vi "SENS_AVER.vi"(0 "VISA IN":refnum<visa-resource-name>, 2 "Average ON/OFF":bool, 5 "error in":errorcluster, 7 "Channel":i32) -> (14 "VISA Out":refnum<visa-resource-name>, 19 "error out":errorcluster)   [LabVIEW 2018, in "PNA-X.lvlib"]
doc: "SENSe<cnum>:AVERage:CLEar \n(Write-only) Clears and restarts averaging of the measurement data. Must also set \nSENS:AVER[:STATe] ON \nParameters \n<cnum> Any existing channel number; if unspecified, value is set to 1. \nExamples SENS:AVER:CLE \nsense2:average:clear \nQuery Syntax Not applicable \nDefault Not applicable"
uses:
  PNA-X.lvlib
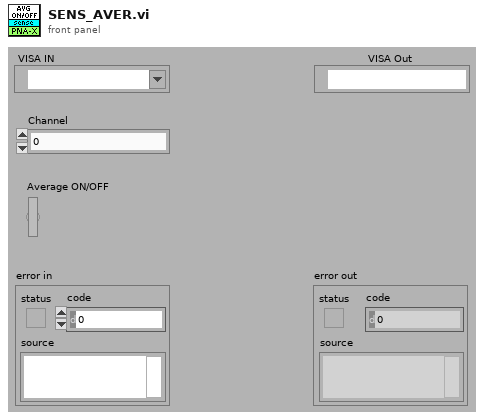
[diagram p1: front panel]
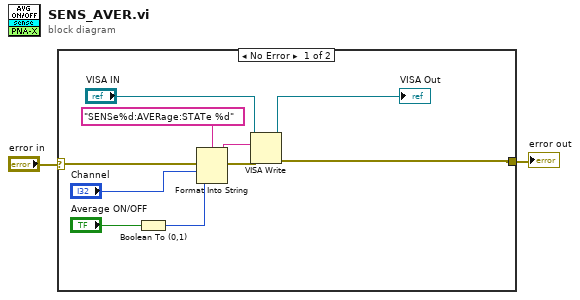
[diagram p0: block diagram]
diagram:
  n1 = case shown="No Error" "error in" {
    selector: "error in" -> [w12 w13]
    tunnel: [w8 w13] -> w1
    frame No Error {
      n2 = Boolean To (0,1)(Boolean="Average ON/OFF") -> (0, 1=w4:i16)
      n3 = Format Into String(format string="SENSe%d:AVERage:STATe %d", error in=w12, "Channel", w4) -> (resulting string=w10:string, error out=w11:errorcluster)  [unwired: 1 in]
      n4 = VISA Write(VISA resource name="VISA IN", write buffer=w10, error in (no error)=w11) -> (VISA resource name out=→"VISA Out":refnum<visa-resource-name>, error out=w8:errorcluster)  [unwired: 1 out]
    }
    frame Error {
    }
  }
  "error out" <- w1
